vi "Calculate Orientation.vi"(10 "Accel":cluster{dbl, dbl, dbl}) -> ()   [LabVIEW 2018]
panel:
  out "Pitch":dbl
  out "Roll":dbl
  out "Z":dbl
  out "Y":dbl
  out "X":dbl
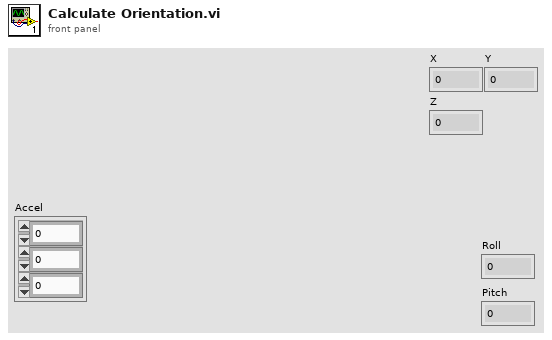
[diagram p1: front panel]
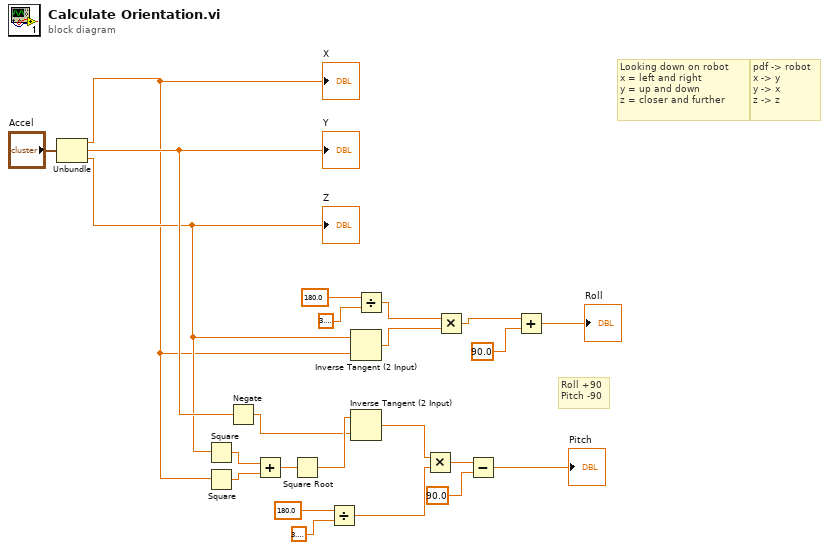
[diagram p0: block diagram]
diagram:
  # "Roll +90\nPitch -90"
  # "pdf -> robot\nx -> y\ny -> x\nz -> z"
  # "Looking down on robot \nx = left and right\ny = up and down\nz = closer and further"
  n1 = Unbundle("Accel") -> (w7:dbl, w9:dbl, w8:dbl)
  "X" <- w7
  "Y" <- w9
  "Z" <- w8
  n2 = Square(x=w8) -> (x^2=w17:dbl)
  n3 = Square(x=w7) -> (x^2=w18:dbl)
  n4 = Negate(x=w9) -> (-x=w10:dbl)
  n5 = Add(x=w17, y=w18) -> (x+y=w16:dbl)
  n6 = Square Root(x=w16) -> (sqrt(x)=w11:dbl)
  n7 = Divide(x=180.0, y=3.141592653589793) -> (x/y=w12:dbl)
  n8 = Inverse Tangent (2 Input)(1:w7, 2:w8) -> (0:w20:dbl)
  n9 = Inverse Tangent (2 Input)(1:w10, 2:w11) -> (0:w13:dbl)
  n10 = Divide(x=180.0, y=3.141592653589793) -> (x/y=w19:dbl)
  n11 = Multiply(x=w13, y=w12) -> (x*y=w4:dbl)
  n12 = Multiply(x=w19, y=w20) -> (x*y=w5:dbl)
  n13 = Subtract(x=w4, y=90.0) -> (x-y=→"Pitch":dbl)
  n14 = Add(x=w5, y=90.0) -> (x+y=→"Roll":dbl)
